vi "GetRID.vi"(8 "Student ID in":i32, 9 "all rows in in":string[][](array[string]), 10 "index":i32=11) -> (1 "Record ID":string)   [LabVIEW 2016]
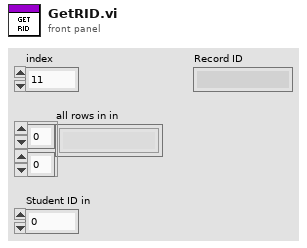
[diagram p1: front panel]
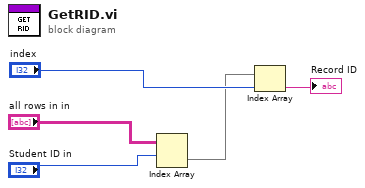
[diagram p0: block diagram]
diagram:
  n1 = Index Array(array="all rows in in", index (row)="Student ID in") -> (element=w3:string[])  [unwired: 1 in]
  n2 = Index Array(array=w3, index="index") -> (element=→"Record ID":string)
